vi "DSF.Engine.Framework.Set Builder Manager.vi"(10 "Builder Manager":refnum<class "DSF.Engine.BuilderManager.lvclass">, 11 "Framework in":refnum<class "Framework.lvclass">) -> (3 "Framework out":refnum<class "Framework.lvclass">)   [LabVIEW 2017, in "DSF.Engine.lvlib" / "Framework.lvclass"]
uses:
  Framework.lvclass
  BuilderManager/DSF.Engine.BuilderManager.lvclass
  Framework.lvclass/Framework.ctl
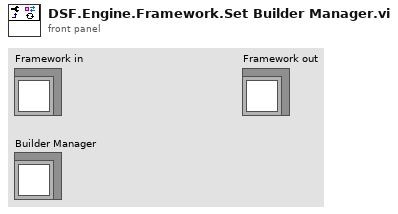
[diagram p1: front panel]
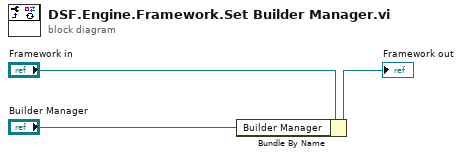
[diagram p0: block diagram]
diagram:
  n1 = Bundle By Name(cluster="Framework in", "Builder Manager"="Builder Manager") -> (→"Framework out":refnum<class "Framework.lvclass">)
